vi "Load to memory.vi"(0 "Py Doc in":refnum<class "Py Doc.lvclass">, 5 "Path":path, 7 "Batch File Path":path, 11 "error in (no error)":errorcluster) -> (4 "Py Doc out":refnum<class "Py Doc.lvclass">, 6 "Names[]":string[](array[string]), 8 "Child Window Data":T1, 15 "error out":errorcluster)   [LabVIEW 2016, in "Py Doc.lvclass"]
uses:
  Py Doc.lvclass
  Private/Child Window Data.ctl
  user32.dll
  LV MDI.lvclass
panel:
  out "hwnd":u32
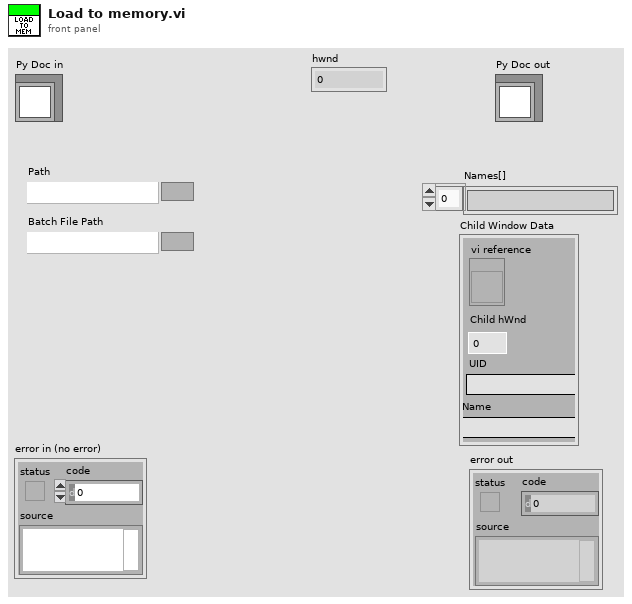
[diagram p1: front panel]
types:
  T1 = typedef "LV MDI.lvclass/Child Window Data.ctl" = cluster{"Child hWnd":u32, "UID":string, "vi reference":refnum<vi>, "Name":string}
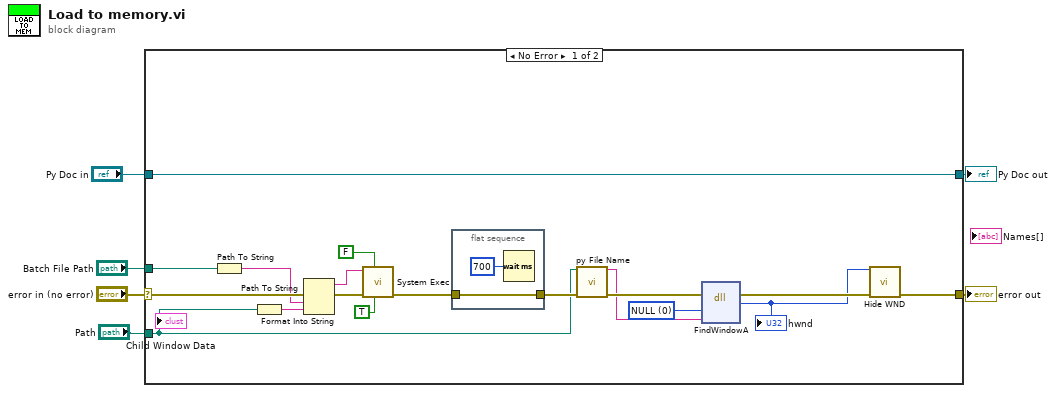
[diagram p0: block diagram]
diagram:
  n1 = case shown="No Error" "error in (no error)" {
    selector: "error in (no error)" -> [w23 w28]
    tunnel: [w15 w28] -> w5
    tunnel: "Py Doc in" -> [w24 w27]
    tunnel: [w24 w27] -> w3
    tunnel: "Path" -> [w7 _]
    tunnel: "Batch File Path" -> [w13 _]
    frame No Error {
      w20 = 0 items=["NULL"]
      n2 = Path To String(path=w13) -> (string=w12:string)
      n3 = Path To String(path=w7) -> (string=w9:string)
      n4 = Format Into String(error in=w23, w12, w9) -> (resulting string=w21:string, error out=w22:errorcluster)  [unwired: 2 in]
      n5 = call <vilib>:"System Exec.vi"("run minimized? (F)"=TRUE, "wait until completion? (T)"=FALSE, "error in (no error)"=w22, "command line"=w21) -> ("error out"=w17:errorcluster)  [unwired: 4 in, 3 out]
      n6 = flat-sequence {
        tunnel: w17 -> [w26]
        tunnel: [w26] -> w10
        frame #0 {
          n7 = Wait (ms)(milliseconds to wait=u32 700) -> ()  [unwired: 1 out]
        }
      }
      n8 = call "py File Name.vi"("Path"=w7, "error in (no error)"=w10) -> ("String"=w8:string, "error out"=w11:errorcluster)  [unwired: 12 in]
      n9 = dll-call lib="user32.dll" fn="FindWindowA"(error in=w11, "lpzsClassName"=w20, "lpzsWindowName"=w8) -> (error out=w16:errorcluster, "hwnd"=w14:u32)  [unwired: 4 in, 1 out]
      "hwnd" <- w14
      n10 = call "Hide WND.vi"("hwnd"=w14, "error in (no error)"=w16) -> ("error out"=w15:errorcluster)  [unwired: 13 in]
    }
    frame Error {
    }
  }
  "error out" <- w5
  "Py Doc out" <- w3
